vi "Factorial.vi"() -> ()   [LabVIEW 2019]
panel:
  out "Input number":i32
  out "Factorial":i32
  in  "stop":bool
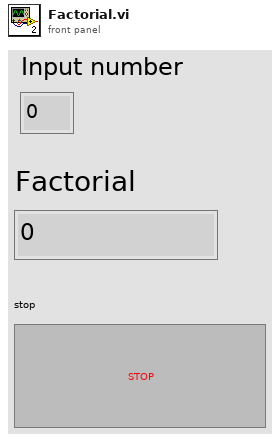
[diagram p1: front panel]
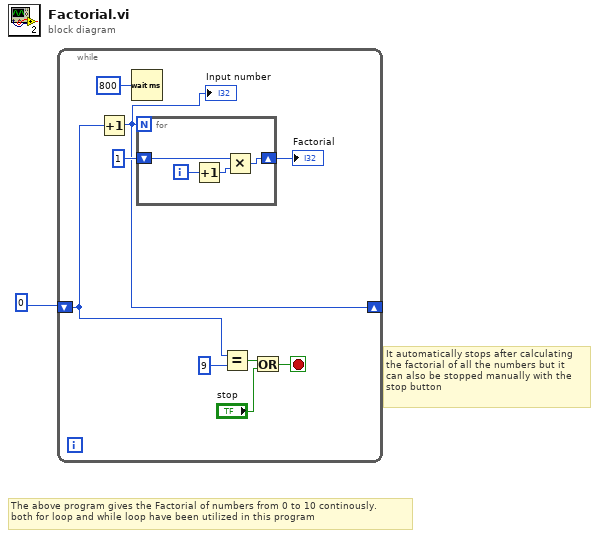
[diagram p0: block diagram]
diagram:
  # "It automatically stops after calculating\nthe factorial of all the numbers but it\ncan also be stopped manually with the\nstop button"
  # "The above program gives the Factorial of numbers from 0 to 10 continously.\nboth for loop and while loop have been utilized in this program"
  n1 = while {
    shift-right: [w2] -> _
    shift-left: 0 -> [w7]
    stop <- w9 stop-if-true
    n2 = Increment(x=w7) -> (x+1=w2:i32)
    "Input number" <- w2
    n3 = Wait (ms)(milliseconds to wait=u32 800) -> ()  [unwired: 1 out]
    n4 = for {
      N: w2 -> [_]
      shift-right: [w11] -> w4
      shift-left: 1 -> [w12]
      i -> [w13]
      n5 = Increment(x=w13) -> (x+1=w14:i32)
      n6 = Multiply(x=w12, y=w14) -> (x*y=w11:i32)
    }
    "Factorial" <- w4
    n7 = Equal?(x=w7, y=9) -> (x = y?=w10:bool)
    n8 = Or(x=w10, y="stop") -> (x .or. y?=w9:bool)
  }
